vi "Update Graphs_JL.vi"(0 "Select Graph":T12, 2 "appended array":refnum<vi>[](array[refnum]), 5 "ERD Graph  Ind 2":T11, 7 "ERD_Data_Bundled_In":T1, 11 "Error In":errorcluster) -> (1 "All Loads":u16[][](graph), 3 "Inlet Thermistor":u16(graph), 4 "Raw Moisture":u16(graph), 6 "Filtered Moisture":u16(graph), 8 "Outlet Thermistor":u16(graph), 12 "ERD 3":dbl(graph), 13 "ERD 2":dbl(graph), 14 "ERD 1":dbl(graph), 15 "Error Out":errorcluster)   [LabVIEW 2023]
doc: "This VI displays (makes visable) the corresponding graph based on user selection, as well as updates the values of the graphs with current data."
uses:
  type defs/Select _Graph_JL.ctl
  type defs/All_Bundled_Data_JL.ctl
  Common/type defs/Version.ctl
  type defs/ERD_Always_Show_JL.ctl
  Common/type defs/CSV_File_String_Arrays.ctl
  Common/type defs/Fault Table Array.ctl
  Common/type defs/Fault_Table_Info.ctl
  type defs/Heat Control.ctl
  type defs/ERD_Commercial_Laundry.ctl
  Common/type defs/BootloaderVersion.ctl
  type defs/ERD_RJ45.ctl
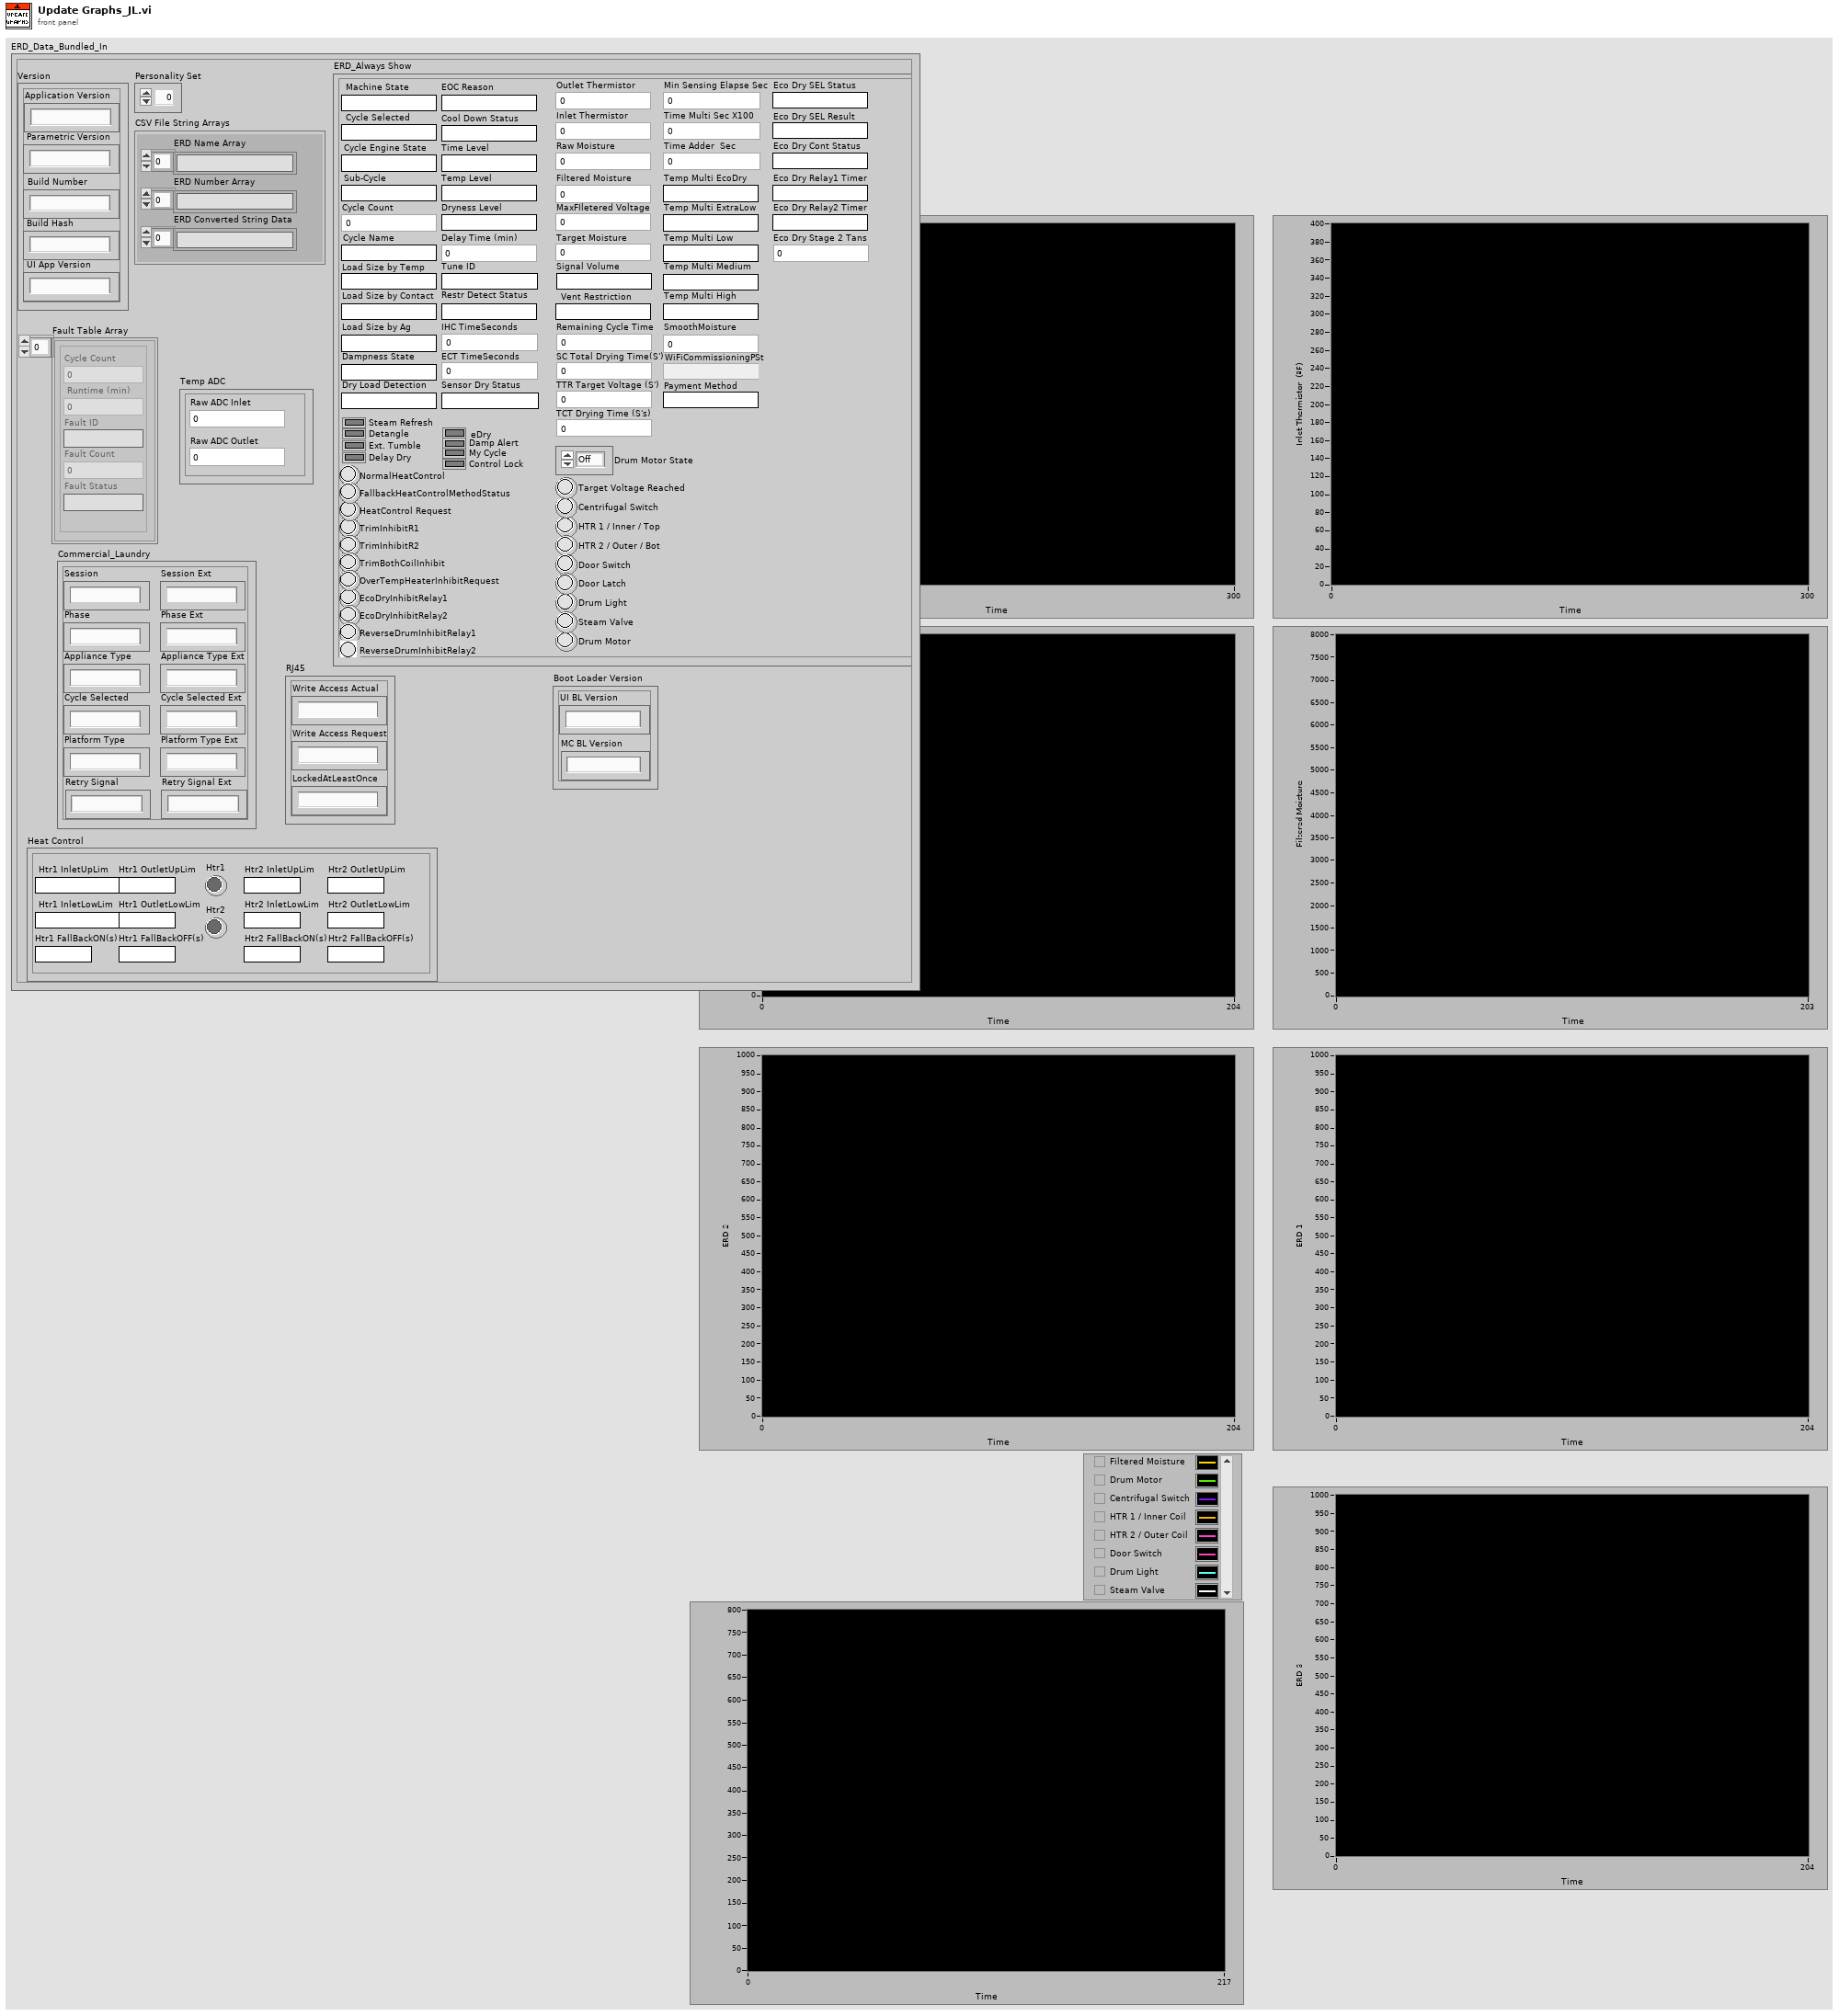
[diagram p1: front panel]
types:
  T1 = typedef "All_Bundled_Data_JL.ctl" = cluster{"Version":T2, "ERD_Always Show":T3, "Personality Set":u8, "CSV File String Arrays":T4, "Fault Table Array ":T5, "Heat Control":T7, "Temp ADC":cluster{"Raw ADC Outlet":u16, "Raw ADC Inlet":u16}, "Commercial_Laundry":T8, "Boot Loader Version":T9, "RJ45":T10}
  T2 = typedef "Version.ctl" = cluster{"Build Number":string, "Build Hash ":string, "Application Version":string, "Parametric Version":string, "UI App Version":string}
  T3 = typedef "ERD_Always_Show_JL.ctl" = cluster{"Inlet Thermistor":u16, "Machine State":string, "Filtered Moisture":u16, "Cycle Selected":string, "HTR 1 / Inner / Top":bool, "HTR 2 / Outer / Bot":bool, "Door Switch":bool, "Drum Light":bool, "Cycle Engine State":string, "Centrifugal Switch":bool, "Drum Motor":bool, "Cycle Count":u32, "Ext. Tumble":bool, "eDry":bool, "Temp Level":string, "Dryness Level":string, "Time Level":string, "Delay Time (min)":u16, "Steam Refresh":bool, "Damp Alert":bool, "Sub-Cycle":string, "Outlet Thermistor":u16, "Target Moisture":u16, "Remaining Cycle Time":u32, "Raw Moisture":u16, "Cycle Name":string, "My Cycle":bool, "Delay Dry":bool, "Detangle":bool, "Control Lock":bool, "Steam Valve":bool, "Door Latch":bool, "Signal Volume":string, "Tune ID":string, "Restr Detect Status":string, "Vent Restriction":string, "Load Size by Contact":string, "Load Size by Temp":string, "EOC Reason":string, "Sensor Dry Status":string, "Dampness State":string, "Target Voltage Reached":bool, "TrimInhibitR1":bool, "TrimInhibitR2":bool, "TrimBothCoilInhibit":bool, "NormalHeatControl":bool, "HeatControl Request":bool, "Cool Down Status":string, "EcoDryInhibitRelay1":bool, "EcoDryInhibitRelay2":bool, "ReverseDrumInhibitRelay1":bool, "ReverseDrumInhibitRelay2":bool, "OverTempHeaterInhibitRequest":bool, "FallbackHeatControlMethodStatus":bool, "IHC TimeSeconds":u32, "ECT TimeSeconds ":u32, "SC Total Drying Time(S')":u32, "TTR Target Voltage (S')":u32, "TCT Drying Time (S's)":u32, "Drum Motor State":enum16{"Off", "Cw", "Ccw", "Max"}, "Load Size by Ag":string, "MaxFIletered Voltage":u16, "Dry Load Detection":string, "Min Sensing Elapse Sec":u32, "Time Multi Sec X100":u32, "Time Adder  Sec":u32, "Temp Multi EcoDry":string, "Temp Multi ExtraLow":string, "Temp Multi Low ":string, "Temp Multi Medium":string, "Temp Multi High":string, "SmoothMoisture":u16, "Eco Dry SEL Status":string, "Eco Dry SEL Result":string, "Eco Dry Cont Status":string, "Eco Dry Relay1 Timer":string, "Eco Dry Relay2 Timer ":string, "Eco Dry Stage 2 Tans ":u32, "WiFiCommissioningPSt":string, "Payment Method":string}
  T4 = typedef "CSV_File_String_Arrays.ctl" = cluster{"ERD Number Array":string[], "ERD Name Array":string[], "ERD Converted String Data":string[]}
  T5 = typedef "Fault Table Array.ctl" = T6[]
  T6 = typedef "Fault_Table_Info.ctl" = cluster{"Cycle Count":u32, " Runtime (min) ":u32, "Fault Status":string, "Fault ID":string, "Fault Count":u16}
  T7 = typedef "Heat Control.ctl" = cluster{"Htr1 InletLowLim":string, "Htr1 InletUpLim":string, "Htr1 OutletLowLim":string, "Htr1 OutletUpLim":string, "Htr1 FallBackON(s)":string, "Htr1 FallBackOFF(s)":string, "Htr1":bool, "Htr2 InletLowLim":string, "Htr2 InletUpLim":string, "Htr2 OutletLowLim":string, "Htr2 OutletUpLim":string, "Htr2 FallBackON(s)":string, "Htr2 FallBackOFF(s)":string, "Htr2":bool}
  T8 = typedef "ERD_Commercial_Laundry.ctl" = cluster{"Session":string, "Phase":string, "Appliance Type":string, "Cycle Selected":string, "Platform Type":string, "Retry Signal":string, "Session Ext":string, "Phase Ext":string, "Appliance Type Ext":string, "Cycle Selected Ext":string, "Platform Type Ext":string, "Retry Signal Ext":string}
  T9 = typedef "BootloaderVersion.ctl" = cluster{"UI BL Version":string, "MC BL Version":string}
  T10 = typedef "ERD_RJ45.ctl" = cluster{"Write Access Actual":string, "Write Access Request":string, "LockedAtLeastOnce":string}
  T11 = cluster{"ERD Value 1":dbl, "ERD Value 2":dbl, "ERD Value 3":dbl}
  T12 = typedef "Select _Graph_JL.ctl" = enum16{"All Loads", "Inlet Thermistor", "Outlet Thermistor", "Raw Moisture", "Filtered Moisture", "ERD 1", "ERD 2", "ERD 3"}
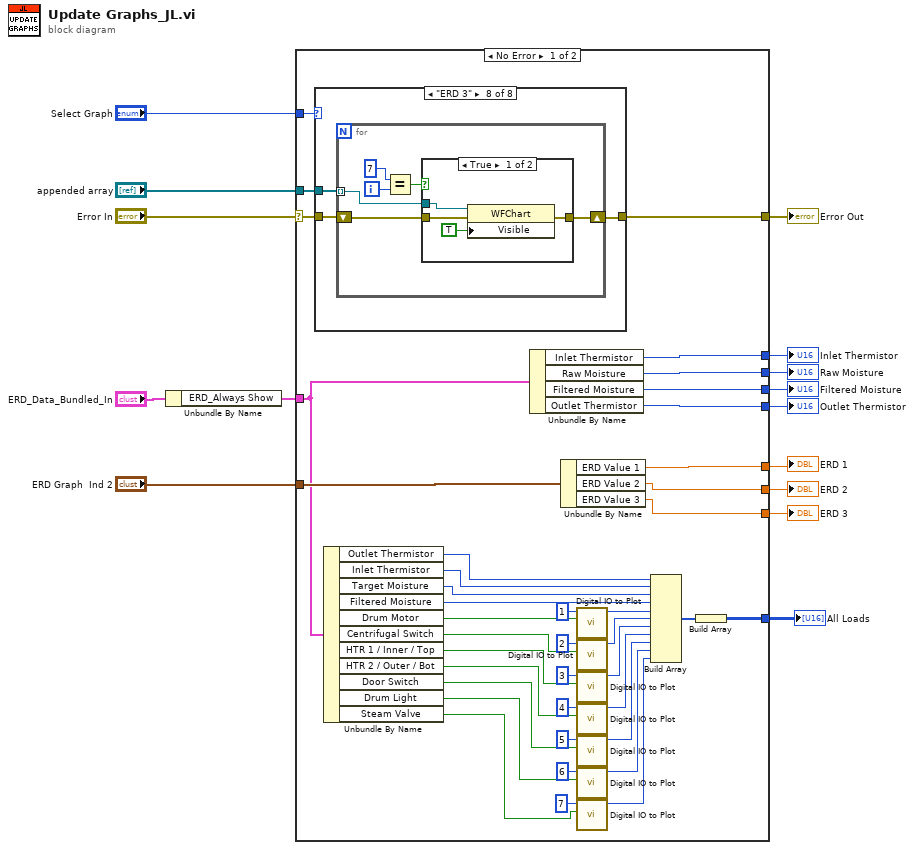
[diagram p0: block diagram]
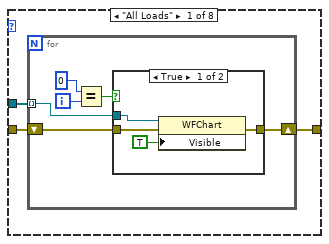
[diagram p2: hidden frame]
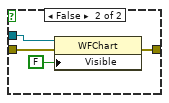
[diagram p3: hidden frame]
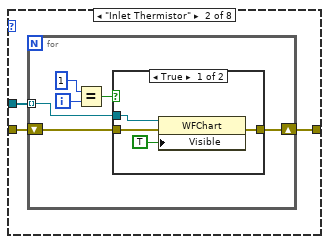
[diagram p4: hidden frame]
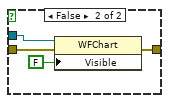
[diagram p5: hidden frame]
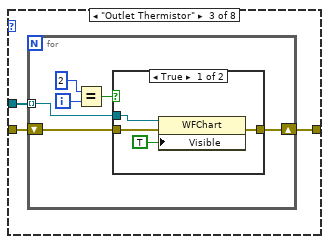
[diagram p6: hidden frame]
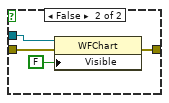
[diagram p7: hidden frame]
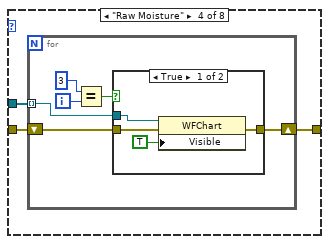
[diagram p8: hidden frame]
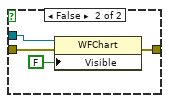
[diagram p9: hidden frame]
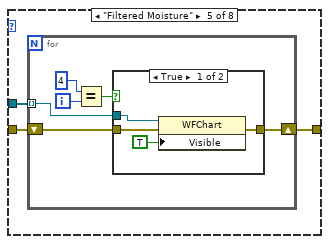
[diagram p10: hidden frame]
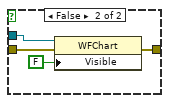
[diagram p11: hidden frame]
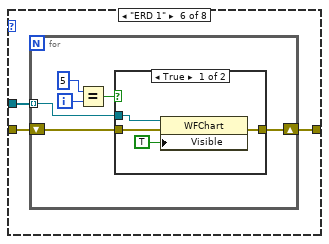
[diagram p12: hidden frame]
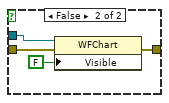
[diagram p13: hidden frame]
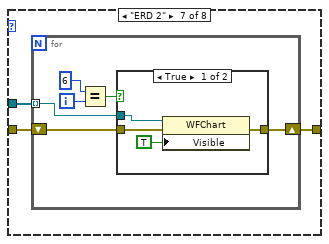
[diagram p14: hidden frame]
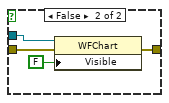
[diagram p15: hidden frame]
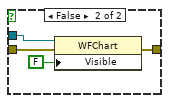
[diagram p16: hidden frame]
diagram:
  n1 = Unbundle By Name("ERD_Data_Bundled_In") -> ("ERD_Always Show"=w4:T3)
  n2 = case shown="No Error" "Error In" {
    selector: "Error In" -> [w53 w192]
    tunnel: [w52 w192] -> w14
    tunnel: w4 -> [w43 _]
    tunnel: "appended array" -> [w54 _]
    tunnel: "Select Graph" -> [w55 _]
    tunnel: [w51 _] -> w11
    tunnel: [w50 _] -> w1
    tunnel: [w49 _] -> w10
    tunnel: [w48 _] -> w9
    tunnel: "ERD Graph  Ind 2" -> [w47 _]
    tunnel: [w46 _] -> w7
    tunnel: [w45 _] -> w6
    tunnel: [w44 _] -> w5
    tunnel: [w19 _] -> w2
    frame No Error {
      n3 = case shown="\"ERD 3\"" w55 {
        tunnel: w54 -> [w58 w75 w92 w109 w125 w142 w160 w175]
        tunnel: w53 -> [w57 w74 w91 w108 w126 w143 w159 w177]
        tunnel: [w56 w73 w90 w107 w124 w141 w158 w176] -> w52
        frame "All Loads" {
          n4 = for {
            tunnel: w58 -> [w64] mode=indexing
            shift-right: [w62] -> w56
            shift-left: w57 -> [w63]
            i -> [w61]
            n5 = Equal?(x=0 ("index"), y=w61) -> (x = y?=w59:bool)
            n6 = case shown="True" w59 {
              tunnel: w64 -> [w68 w72]
              tunnel: w63 -> [w66 w70]
              tunnel: [w65 w69] -> w62
              frame True {
                n7 = property class="WFChart"(reference=w68, error in=w66, "Visible"=TRUE) -> (error out=w65:errorcluster)  [unwired: 1 out]
              }
              frame False {
                n8 = property class="WFChart"(reference=w72, error in=w70, "Visible"=FALSE) -> (error out=w69:errorcluster)  [unwired: 1 out]
              }
            }
          }
        }
        frame "Inlet Thermistor" {
          n9 = for {
            tunnel: w75 -> [w81] mode=indexing
            shift-right: [w79] -> w73
            shift-left: w74 -> [w80]
            i -> [w78]
            n10 = Equal?(x=1 ("index"), y=w78) -> (x = y?=w76:bool)
            n11 = case shown="True" w76 {
              tunnel: w81 -> [w85 w89]
              tunnel: w80 -> [w83 w87]
              tunnel: [w82 w86] -> w79
              frame True {
                n12 = property class="WFChart"(reference=w85, error in=w83, "Visible"=TRUE) -> (error out=w82:errorcluster)  [unwired: 1 out]
              }
              frame False {
                n13 = property class="WFChart"(reference=w89, error in=w87, "Visible"=FALSE) -> (error out=w86:errorcluster)  [unwired: 1 out]
              }
            }
          }
        }
        frame "Outlet Thermistor" {
          n14 = for {
            tunnel: w92 -> [w98] mode=indexing
            shift-right: [w96] -> w90
            shift-left: w91 -> [w97]
            i -> [w95]
            n15 = Equal?(x=2 ("index"), y=w95) -> (x = y?=w93:bool)
            n16 = case shown="True" w93 {
              tunnel: w98 -> [w102 w106]
              tunnel: w97 -> [w100 w104]
              tunnel: [w99 w103] -> w96
              frame True {
                n17 = property class="WFChart"(reference=w102, error in=w100, "Visible"=TRUE) -> (error out=w99:errorcluster)  [unwired: 1 out]
              }
              frame False {
                n18 = property class="WFChart"(reference=w106, error in=w104, "Visible"=FALSE) -> (error out=w103:errorcluster)  [unwired: 1 out]
              }
            }
          }
        }
        frame "Raw Moisture" {
          n19 = for {
            tunnel: w109 -> [w115] mode=indexing
            shift-right: [w113] -> w107
            shift-left: w108 -> [w114]
            i -> [w112]
            n20 = Equal?(x=3 ("index"), y=w112) -> (x = y?=w110:bool)
            n21 = case shown="True" w110 {
              tunnel: w115 -> [w119 w123]
              tunnel: w114 -> [w117 w121]
              tunnel: [w116 w120] -> w113
              frame True {
                n22 = property class="WFChart"(reference=w119, error in=w117, "Visible"=TRUE) -> (error out=w116:errorcluster)  [unwired: 1 out]
              }
              frame False {
                n23 = property class="WFChart"(reference=w123, error in=w121, "Visible"=FALSE) -> (error out=w120:errorcluster)  [unwired: 1 out]
              }
            }
          }
        }
        frame "Filtered Moisture" {
          n24 = for {
            tunnel: w125 -> [w132] mode=indexing
            shift-right: [w130] -> w124
            shift-left: w126 -> [w131]
            i -> [w129]
            n25 = Equal?(x=4 ("index"), y=w129) -> (x = y?=w127:bool)
            n26 = case shown="True" w127 {
              tunnel: w132 -> [w136 w140]
              tunnel: w131 -> [w134 w138]
              tunnel: [w133 w137] -> w130
              frame True {
                n27 = property class="WFChart"(reference=w136, error in=w134, "Visible"=TRUE) -> (error out=w133:errorcluster)  [unwired: 1 out]
              }
              frame False {
                n28 = property class="WFChart"(reference=w140, error in=w138, "Visible"=FALSE) -> (error out=w137:errorcluster)  [unwired: 1 out]
              }
            }
          }
        }
        frame "ERD 1" {
          n29 = for {
            tunnel: w142 -> [w149] mode=indexing
            shift-right: [w147] -> w141
            shift-left: w143 -> [w148]
            i -> [w146]
            n30 = Equal?(x=5 ("index"), y=w146) -> (x = y?=w144:bool)
            n31 = case shown="True" w144 {
              tunnel: w149 -> [w153 w157]
              tunnel: w148 -> [w151 w155]
              tunnel: [w150 w154] -> w147
              frame True {
                n32 = property class="WFChart"(reference=w153, error in=w151, "Visible"=TRUE) -> (error out=w150:errorcluster)  [unwired: 1 out]
              }
              frame False {
                n33 = property class="WFChart"(reference=w157, error in=w155, "Visible"=FALSE) -> (error out=w154:errorcluster)  [unwired: 1 out]
              }
            }
          }
        }
        frame "ERD 2" {
          n34 = for {
            tunnel: w160 -> [w166] mode=indexing
            shift-right: [w164] -> w158
            shift-left: w159 -> [w165]
            i -> [w163]
            n35 = Equal?(x=6 ("index"), y=w163) -> (x = y?=w161:bool)
            n36 = case shown="True" w161 {
              tunnel: w166 -> [w170 w174]
              tunnel: w165 -> [w168 w172]
              tunnel: [w167 w171] -> w164
              frame True {
                n37 = property class="WFChart"(reference=w170, error in=w168, "Visible"=TRUE) -> (error out=w167:errorcluster)  [unwired: 1 out]
              }
              frame False {
                n38 = property class="WFChart"(reference=w174, error in=w172, "Visible"=FALSE) -> (error out=w171:errorcluster)  [unwired: 1 out]
              }
            }
          }
        }
        frame "ERD 3" {
          n39 = for {
            tunnel: w175 -> [w183] mode=indexing
            shift-right: [w181] -> w176
            shift-left: w177 -> [w182]
            i -> [w180]
            n40 = Equal?(x=7 ("index"), y=w180) -> (x = y?=w178:bool)
            n41 = case shown="True" w178 {
              tunnel: w183 -> [w187 w191]
              tunnel: w182 -> [w185 w189]
              tunnel: [w184 w188] -> w181
              frame True {
                n42 = property class="WFChart"(reference=w187, error in=w185, "Visible"=TRUE) -> (error out=w184:errorcluster)  [unwired: 1 out]
              }
              frame False {
                n43 = property class="WFChart"(reference=w191, error in=w189, "Visible"=FALSE) -> (error out=w188:errorcluster)  [unwired: 1 out]
              }
            }
          }
        }
      }
      n44 = Unbundle By Name(w43) -> ("Outlet Thermistor"=w16:u16, "Inlet Thermistor"=w17:u16, "Target Moisture"=w18:u16, "Filtered Moisture"=w42:u16, "Drum Motor"=w41:bool, "Centrifugal Switch"=w39:bool, "HTR 1 / Inner / Top"=w37:bool, "HTR 2 / Outer / Bot"=w35:bool, "Door Switch"=w33:bool, "Drum Light"=w31:bool, "Steam Valve"=w29:bool)
      n45 = Unbundle By Name(w43) -> ("Inlet Thermistor"=w51:u16, "Raw Moisture"=w50:u16, "Filtered Moisture"=w49:u16, "Outlet Thermistor"=w48:u16)
      n46 = Unbundle By Name(w47) -> ("ERD Value 1"=w46:dbl, "ERD Value 2"=w45:dbl, "ERD Value 3"=w44:dbl)
      n47 = call "Digital IO to Plot.vi"("Boolean Value"=w41, "Multiplier"=u16 1) -> ("Output"=w27:u16)  [unwired: 9 in]
      n48 = call "Digital IO to Plot.vi"("Boolean Value"=w39, "Multiplier"=u16 2) -> ("Output"=w26:u16)  [unwired: 9 in]
      n49 = call "Digital IO to Plot.vi"("Boolean Value"=w37, "Multiplier"=u16 3) -> ("Output"=w25:u16)  [unwired: 9 in]
      n50 = call "Digital IO to Plot.vi"("Boolean Value"=w35, "Multiplier"=u16 4) -> ("Output"=w24:u16)  [unwired: 9 in]
      n51 = call "Digital IO to Plot.vi"("Boolean Value"=w33, "Multiplier"=u16 5) -> ("Output"=w23:u16)  [unwired: 9 in]
      n52 = call "Digital IO to Plot.vi"("Boolean Value"=w31, "Multiplier"=u16 6) -> ("Output"=w22:u16)  [unwired: 9 in]
      n53 = call "Digital IO to Plot.vi"("Boolean Value"=w29, "Multiplier"=u16 7) -> ("Output"=w21:u16)  [unwired: 9 in]
      n54 = Build Array(w16, w17, w18, w42, w27, w26, w25, w24, w23, w22, w21) -> (w20:u16[])
      n55 = Build Array(w20) -> (w19:u16[][])
    }
    frame Error {
    }
  }
  "Error Out" <- w14
  "Inlet Thermistor" <- w11
  "Raw Moisture" <- w1
  "Filtered Moisture" <- w10
  "Outlet Thermistor" <- w9
  "ERD 1" <- w7
  "ERD 2" <- w6
  "ERD 3" <- w5
  "All Loads" <- w2
